vi "checkIsInsideContainer.vi"(8 "error in":errorcluster, 10 "ObservableValue":variant, 11 "ObservableName":string) -> (0 "error out":errorcluster, 2 "ObservableValue out":variant[](array[variant]), 3 "ObservableName out":string[](array[string]))   [LabVIEW 2025, in "ObserverClass.lvlib"]
uses:
  ObserverClass.lvlib
  <vilib>/Utility/Data Type/NI_Data Type.lvlib
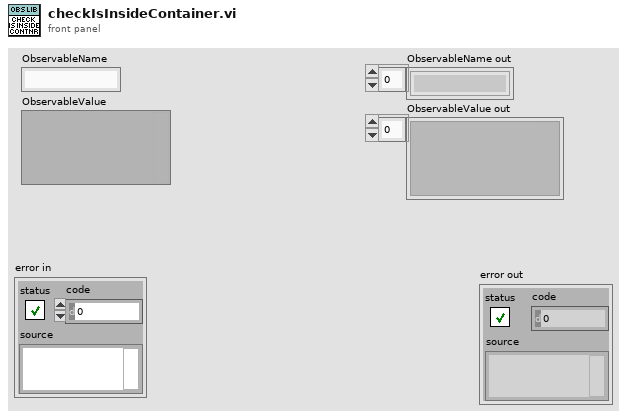
[diagram p1: front panel]
types:
  T1 = enum16{"Get", "Set", "Init", "Remove", "Destroy"}
  T2 = map{string, cluster{"ObserverEvent":refnum<user-event>, "ObserverNr":u64, "Value":variant}}
  T3 = typedef "NI_Data Type.lvlib/Data Type.ctl" = enum8{"Invalid Type", "Void", "I8", "I16", "I32", "I64", "U8", "U16", "U32", "U64", "Single Float", "Double Float", "Extended Float", "Single Complex", "Double Complex", "Extended Complex", "Enum U8", "Enum U16", "Enum U32", "Enum U64", "Single Float With Unit", "Double Float With Unit", "Extended Float With Unit", "Single Complex with Unit", "Double Complex with Unit", "Extended Complex with Unit", "Boolean", "String", "Path", "Picture", "Tag", "Array", "Cluster", "Variant", "LV Variant", "Waveform", "Timestamp", "Digital Waveform", "Digital Data", "ExpressData", "Refnum", "External Data", "VI", "Poly VI", "LabVIEW Class Instance", "Fixed Point", "Set Collection", "Map Collection"}
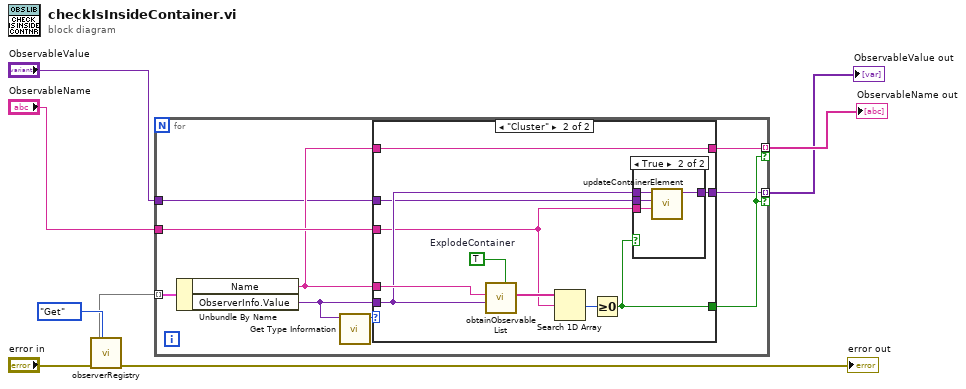
[diagram p0: block diagram]
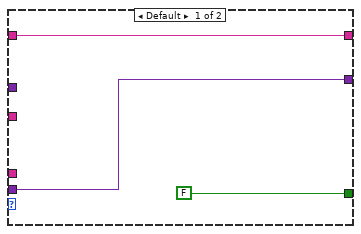
[diagram p2: hidden frame]
diagram:
  n1 = call "observerRegistry.vi"("Action"=T1."Get", "error in"="error in") -> ("error out"=→"error out":errorcluster, "Observable out"=w5:T2)  [unwired: 7 in, 1 out]
  n2 = for {
    tunnel: w5 -> [w16] mode=indexing
    tunnel: [w12] -> w4 mode=indexing if=w15
    tunnel: [w10] -> w3 mode=indexing if=w15
    tunnel: "ObservableName" -> [w14]
    tunnel: "ObservableValue" -> [w9]
    n3 = Unbundle By Name(w16) -> ("Name"=w11:string, "ObserverInfo.Value"=w13:variant)
    n4 = call <vilib>:"Get Type Information.vi"("variant"=w13) -> ("type"=w17:T3)  [unwired: 6 in, 4 out]
    n5 = case shown="\"Cluster\"" w17 {
      tunnel: [FALSE w21] -> w15
      tunnel: w14 -> [_ w23]
      tunnel: w11 -> [_ w30]
      tunnel: w13 -> [w19 w24]
      tunnel: [w18 w26] -> w12
      tunnel: w11 -> [w18 w26]
      tunnel: [w19 w25] -> w10
      tunnel: w9 -> [_ w22]
      frame Default {
      }
      frame "Cluster" {
        w29 = TRUE  # ExplodeContainer
        n6 = call "obtainObservableList.vi"("ExplodeContainer (F)"=w29, "ObservableData"=w24, "ObservableName"=w30) -> ("ObservableName"=w28:string[])  [unwired: 6 in, 2 out]
        n7 = Search 1D Array(1D array=w28, element=w23) -> (index of element=w27:i32)  [unwired: 1 in]
        n8 = Greater Or Equal To 0?(x=w27) -> (x >= 0?=w21:bool)
        n9 = case shown="True" w21 {
          tunnel: [w31 w35] -> w25
          tunnel: w24 -> [w31 w34]
          tunnel: w23 -> [_ w33]
          tunnel: w22 -> [_ w32]
          frame False {
          }
          frame True {
            n10 = call "updateContainerElement.vi"("elementName"=w33, "elementValue"=w32, "Container in"=w34) -> ("Container out"=w35:variant)  [unwired: 8 in]
          }
        }
      }
    }
  }
  "ObservableName out" <- w4
  "ObservableValue out" <- w3
